vi "流量计.vi"() -> ()   [LabVIEW 2016, in "流量计集成.lvlib"]
uses:
  <vilib>/Plasmionique/MB Master/MB_Master_Serial/MB_Master_Serial.lvclass
  C:/Program Files (x86)/National Instruments/LabVIEW 2016/vi.lib/Plasmionique/MB Master/MB_Master/MB_Master.lvclass
  <vilib>/Analysis/baseanly.llb/Mean (DBL).vi
  <vilib>/Utility/config.llb/NI_LVConfig.lvlib
  <vilib>/Analysis/NI_AALBase.lvlib
panel:
  in  "LSS-100X状态查询":bool
  out "流量计通讯 7":bool caption="通讯"
  out "流量计通讯 6":bool caption="通讯"
  out "流量计通讯 5":bool caption="通讯"
  out "流量计通讯 4":bool caption="通讯"
  out "流量计通讯 3":bool caption="通讯"
  out "流量计通讯 2":bool caption="通讯"
  out "流量计通讯":bool caption="通讯"
  in  "baud rate":u32(ring)=9600 caption="波特率" items=["1200"=1200, "2400"=2400, "4800"=4800, "9600"=9600, "19200"=19200, "38400"=38400, "115200"=115200]
  in  "流量计启用 7":bool
  out "流量计类型 7":T1=enum."LS-H600流量计"
  in  "每小时总流量/总累积流量":bool
  out "通信":bool
  in  "释放串口":bool
  in  "打开串口":bool
  out "serial port":refnum<visa-resource-name>="COM10" caption="串口"
  in  "流量计启用 6":bool
  in  "数量 6":u16
  out "流量计类型 6":T1=enum."LSS-100X流量计"
  in  "运行模式":enum16{"按周期模式", "全常规模式"}(ring)=enum."全常规模式"
  in  "流量计启用 5":bool
  in  "数量 5":u16
  out "流量计类型 5":T1=enum."WL1A1明渠流量计"
  in  "流量计启用 4":bool
  in  "数量 4":u16
  out "流量计类型 4":T1=enum."LSH10-1QC流量计"
  out "平均水位":dbl format="%#.2f"
  out "总累积流量":dbl format="%#.2f"
  out "平均流速":dbl format="%#.2f"
  out "总流量":dbl format="%#.2f"
  in  "选项卡控件":T2(tab)
  out "数组":T3[](array[typedef])
  out "数组 2":T4[](array[typedef]) {"累积流量单位" items=["L", "M3", "T", "USG"]; "瞬时流量单位" items=["L/S", "L/M", "L/H", "M3/S", "M3/M", "M3/H", "T/S", "T/M", "T/H", "GPS", "GPM", "GPH"]}
  out "数组 3":T7[](array[typedef])
  out "数组 4":T3[](array[typedef])
  out "数组 5":T3[](array[typedef])
  out "数组 6":T3[](array[typedef])
  out "数组 7":T3[](array[typedef])
  out "MB_Serial session":refnum<class "MB_Master_Serial.lvclass">
  in  "斯坦道功率测流":bool
  in  "流量计启用 3":bool
  in  "数量 3":u16
  out "流量计类型 3":T1=enum."斯坦道功率测流"
  in  "流量计启用 2":bool
  in  "数量 2":u16
  out "流量计类型 2":T1=enum."MGG/KL QC"
  in  "数量":u16
  out "流量计类型":T1
  in  "流量计启用":bool
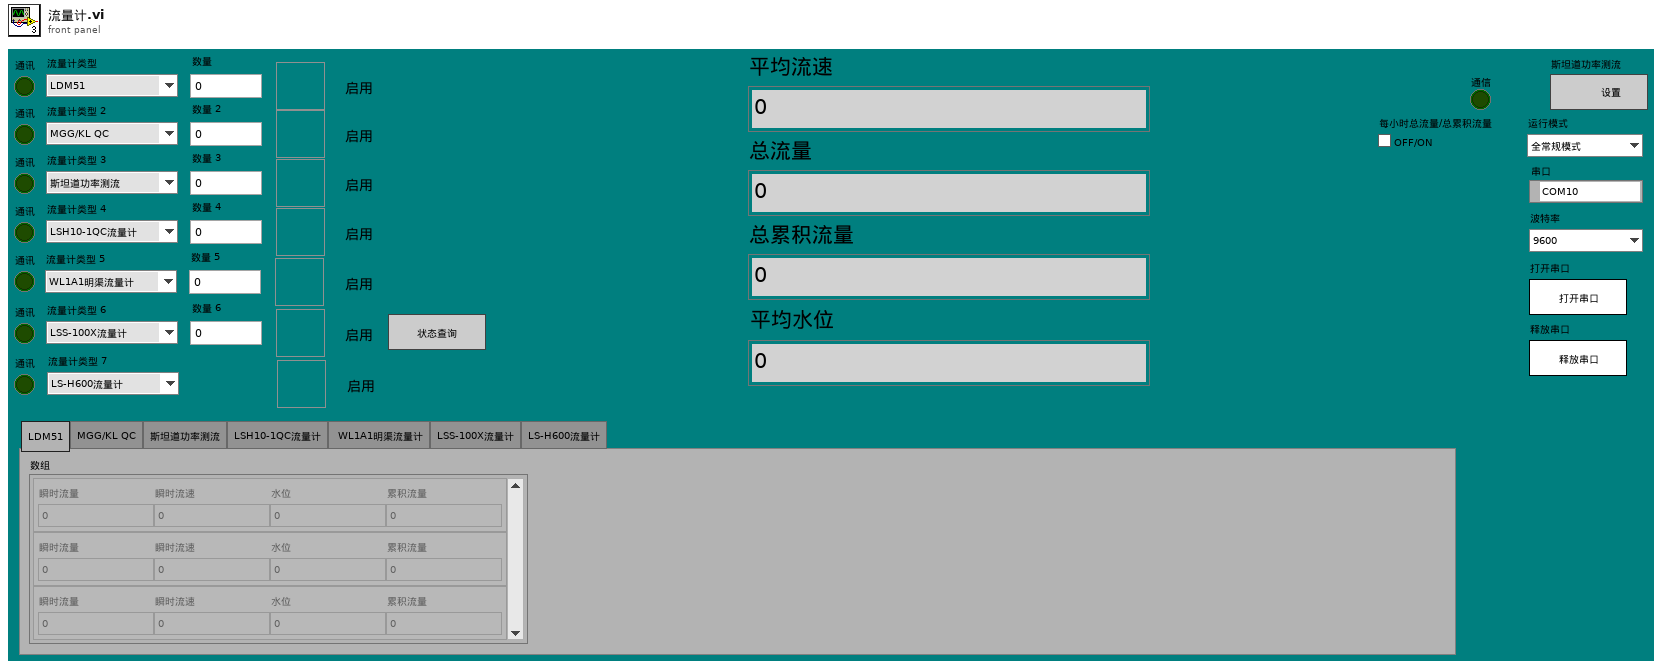
[diagram p1: front panel]
types:
  T1 = typedef "流量计集成.lvlib/流量计类型.ctl" = enum16{"LDM51", "MGG/KL QC", "斯坦道功率测流", "LSH10-1QC流量计", "SL1500-3G", "WL1A1明渠流量计", "LSS-100X流量计", "LS-H600流量计"}
  T2 = enum32{"LDM51", "MGG/KL QC", "斯坦道功率测流", "LSH10-1QC流量计", " WL1A1明渠流量计", "LSS-100X流量计", "LS-H600流量计"}
  T3 = typedef "流量计集成.lvlib/LDM51明渠流量计.lvlib/读取值.ctl" = cluster{"瞬时流量":sgl, "瞬时流速":sgl, "水位":sgl, "累积流量":sgl}
  T4 = typedef "流量计集成.lvlib/MGG-KL-QC流量计.lvlib/读取值.ctl" = cluster{"瞬时流量":sgl, "瞬时流速":sgl, "流量百分比":sgl, "流体电导比":sgl, "正向累积数值":sgl, "反向累积数值":sgl, "瞬时流量单位":T5, "累积流量单位":T6, "上限报警":u16, "下限报警":u16, "空管报警":u16, "系统报警":u16}
  T5 = typedef "流量计集成.lvlib/MGG-KL-QC流量计.lvlib/瞬时流量单位.ctl" = u16
  T6 = typedef "流量计集成.lvlib/MGG-KL-QC流量计.lvlib/累积流量单位.ctl" = u16
  T7 = typedef "流量计集成.lvlib/斯坦道功率测流.lvlib/状态值.ctl" = cluster{"1号瞬时流量":dbl, "2号瞬时流量":dbl, "3号瞬时流量":dbl, "4号瞬时流量":dbl, "5号瞬时流量":dbl, "6号瞬时流量":dbl, "1号累积流量":dbl, "2号累积流量":dbl, "3号累积流量":dbl, "4号累积流量":dbl, "5号累积流量":dbl, "6号累积流量":dbl, "总瞬时流量":dbl, "总累积流量":dbl}
  T8 = typedef "NI_LVConfig.lvlib/Config Data RefNum.ctl" = refnum<k1>
  T9 = cluster{"时间标识":timestamp, "测量模式":string, "数据类型":string, "监测值":sgl, "单位":string, "数据标识":string, "因子编码":string}
  T10 = typedef "LVDateTimeRec.ctl" = cluster{"秒数的小数部分":dbl, "秒":i32, "分":i32, "时":i32, "日":i32, "月":i32, "年":i32, "天数（周）":i32, "天数（年）":i32, "DST":i32}
  T11 = typedef "流量计集成.lvlib/博意达流量计.lvlib/读取值.ctl" = cluster{"瞬时流量":sgl, "瞬时流速":sgl, "水位":sgl, "累积流量":sgl}
  T12 = typedef "流量计集成.lvlib/LSS-100X流量计.lvlib/读取值.ctl" = cluster{"瞬时流量":sgl, "瞬时流速":sgl, "水位":sgl, "累积流量":i32}
  T13 = typedef "流量计集成.lvlib/LS-H600流量计.lvlib/读取值.ctl" = cluster{"瞬时流量":sgl, "瞬时流速":sgl, "水位":sgl, "累积流量":i32}
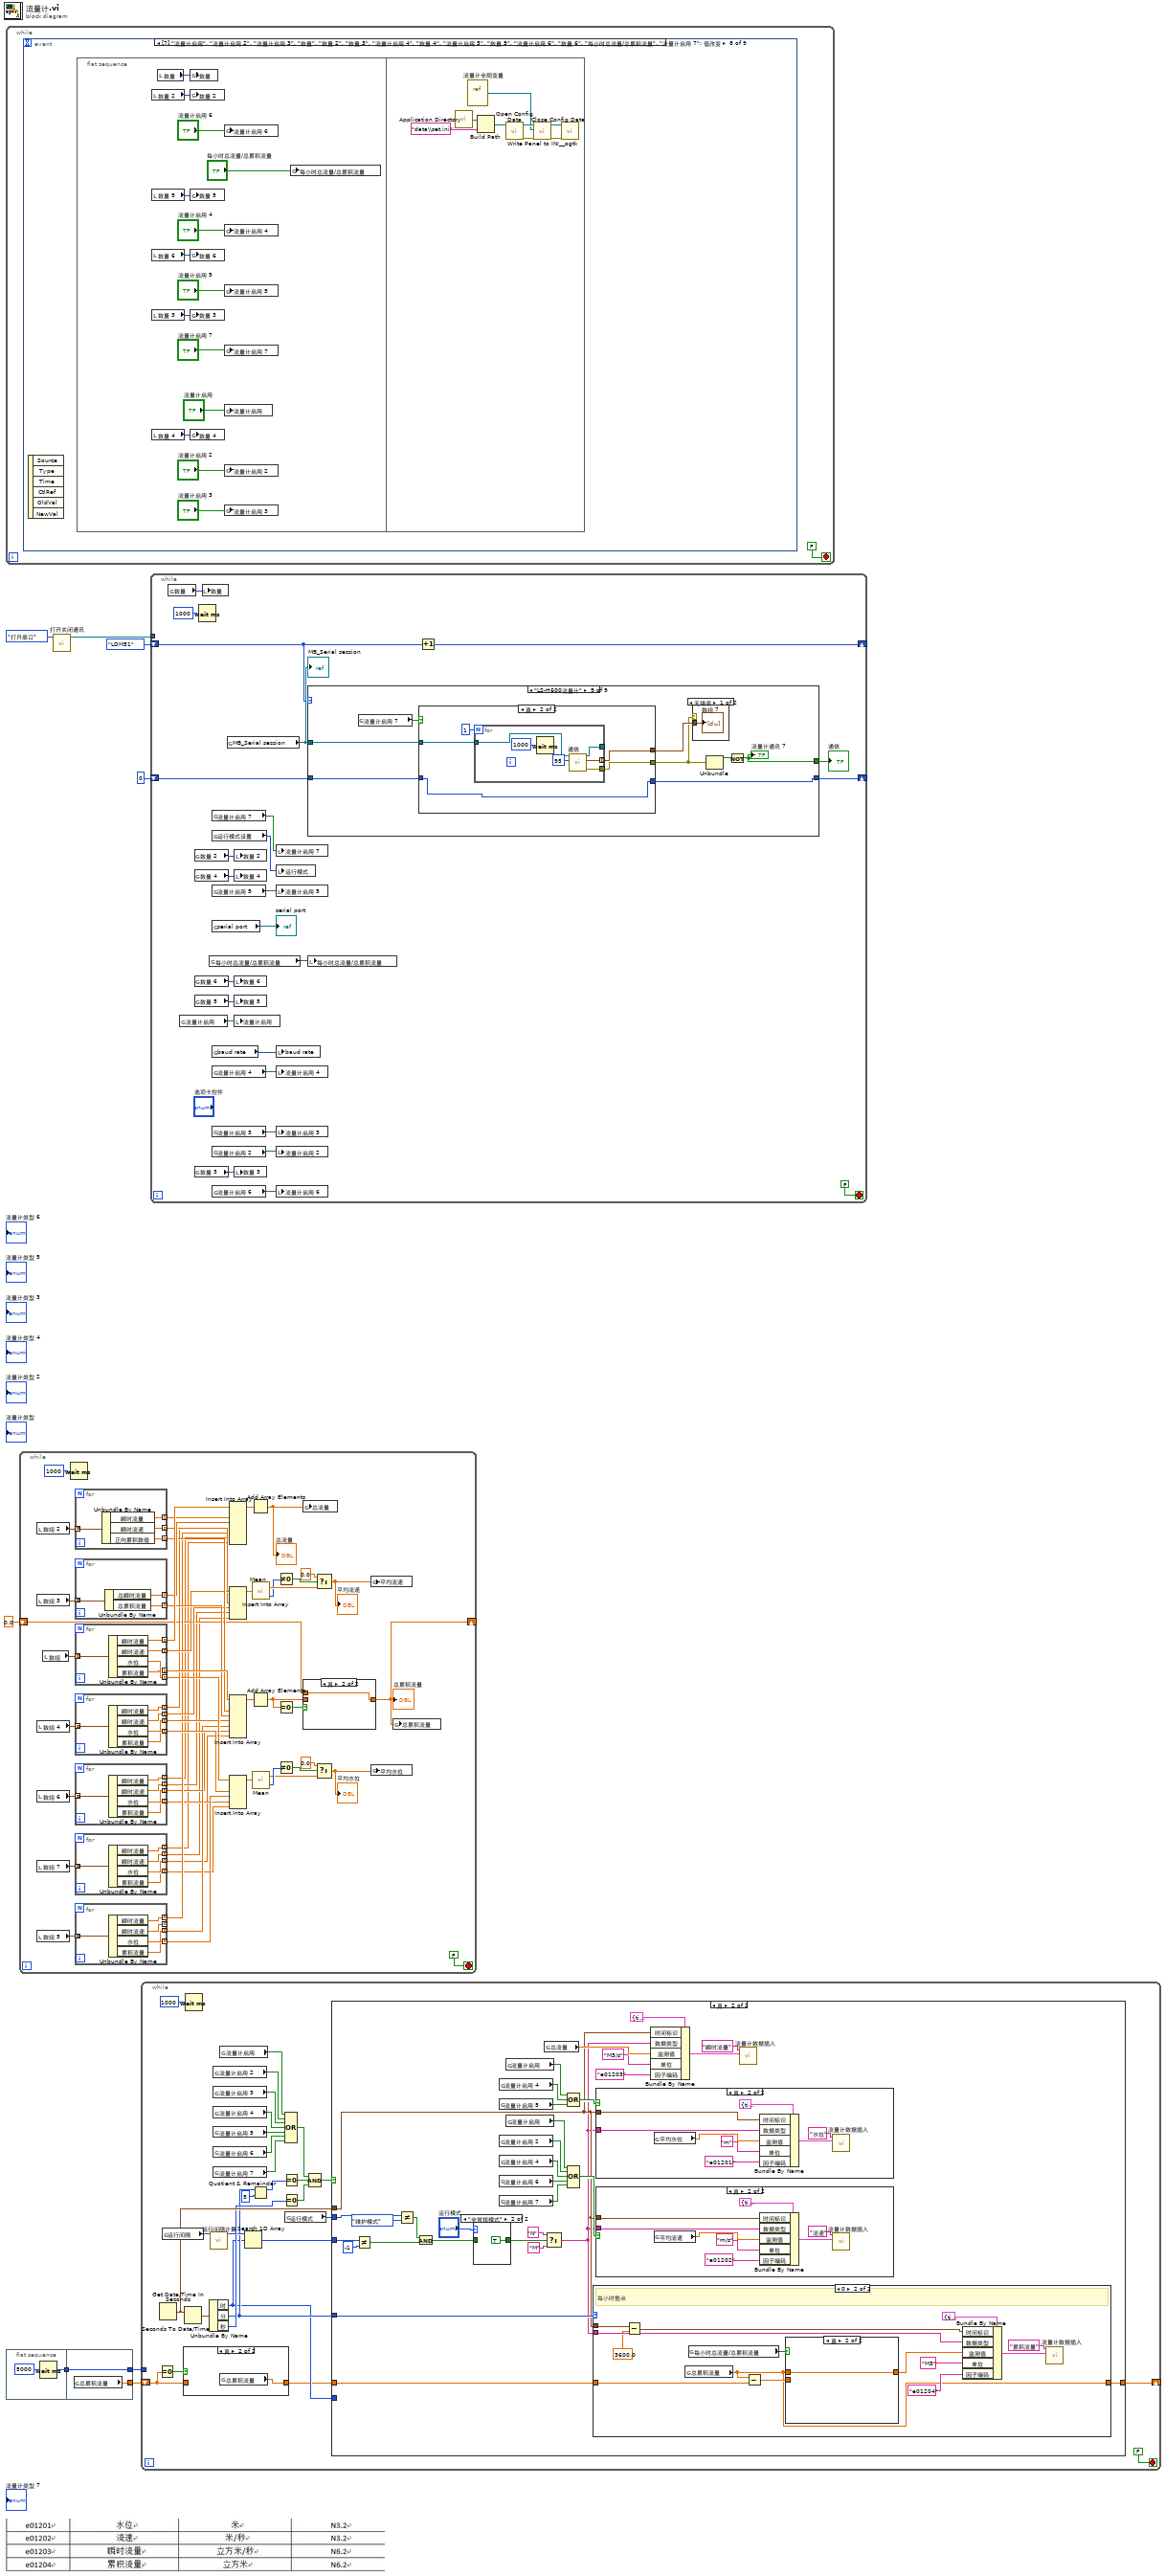
[diagram p0: block diagram]
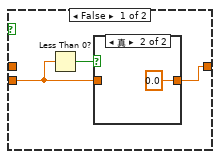
[diagram p6: hidden frame]
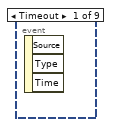
[diagram p11: hidden frame]
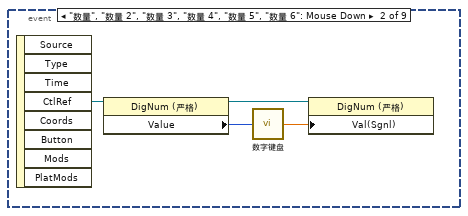
[diagram p12: hidden frame]
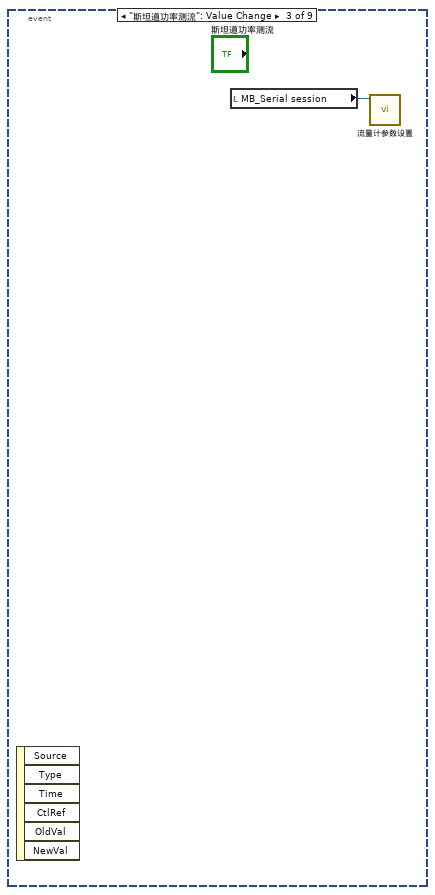
[diagram p13: hidden frame]
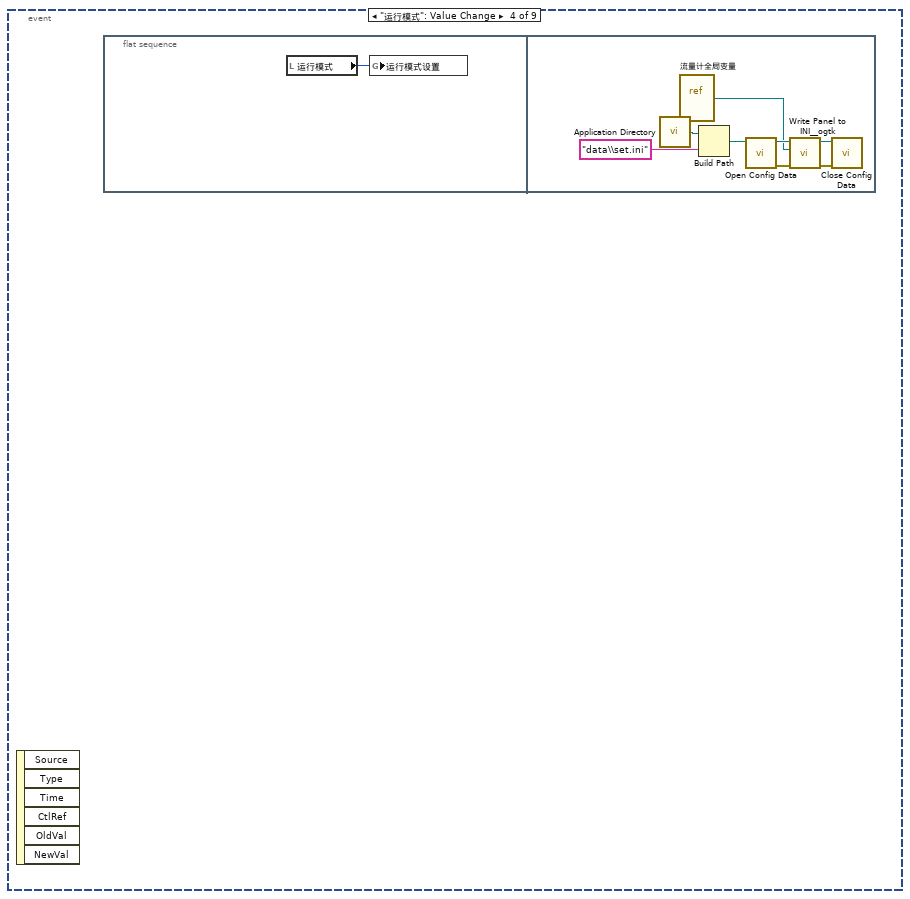
[diagram p14: hidden frame]
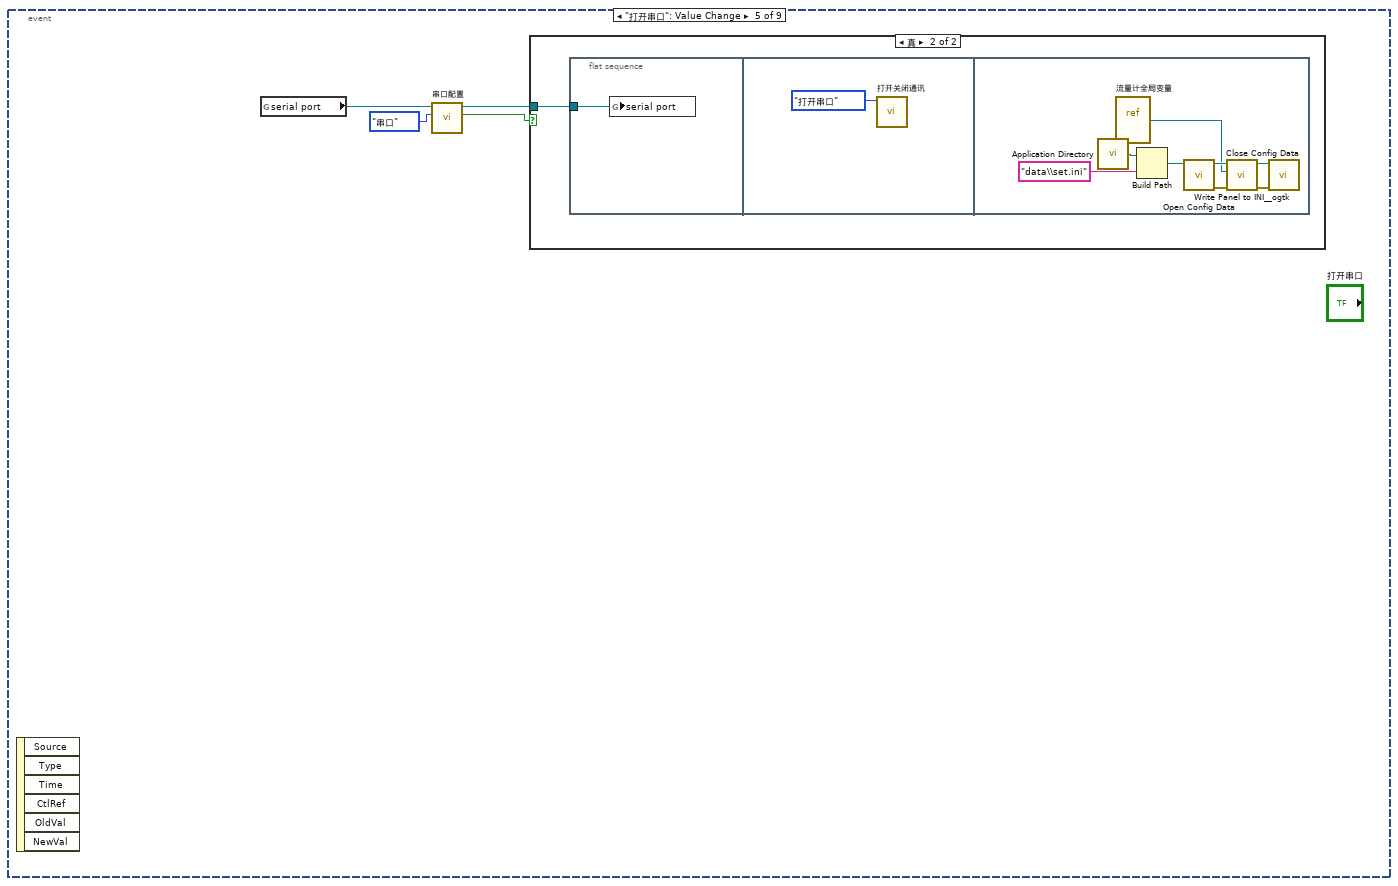
[diagram p15: hidden frame]
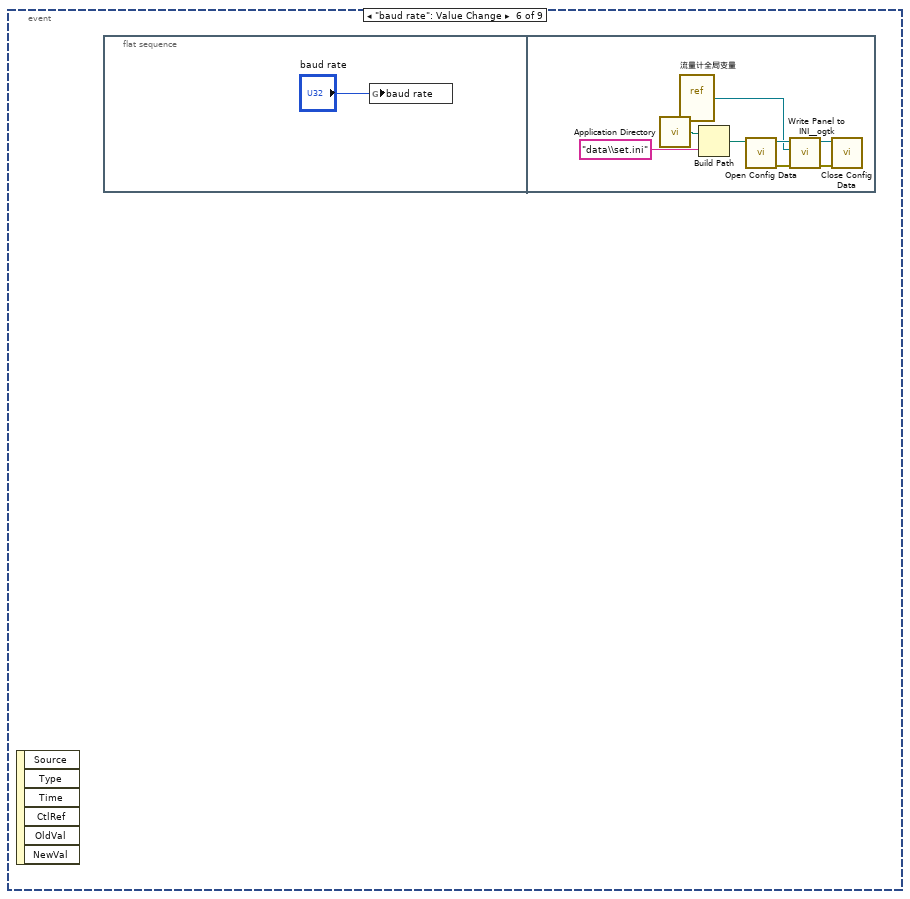
[diagram p17: hidden frame]
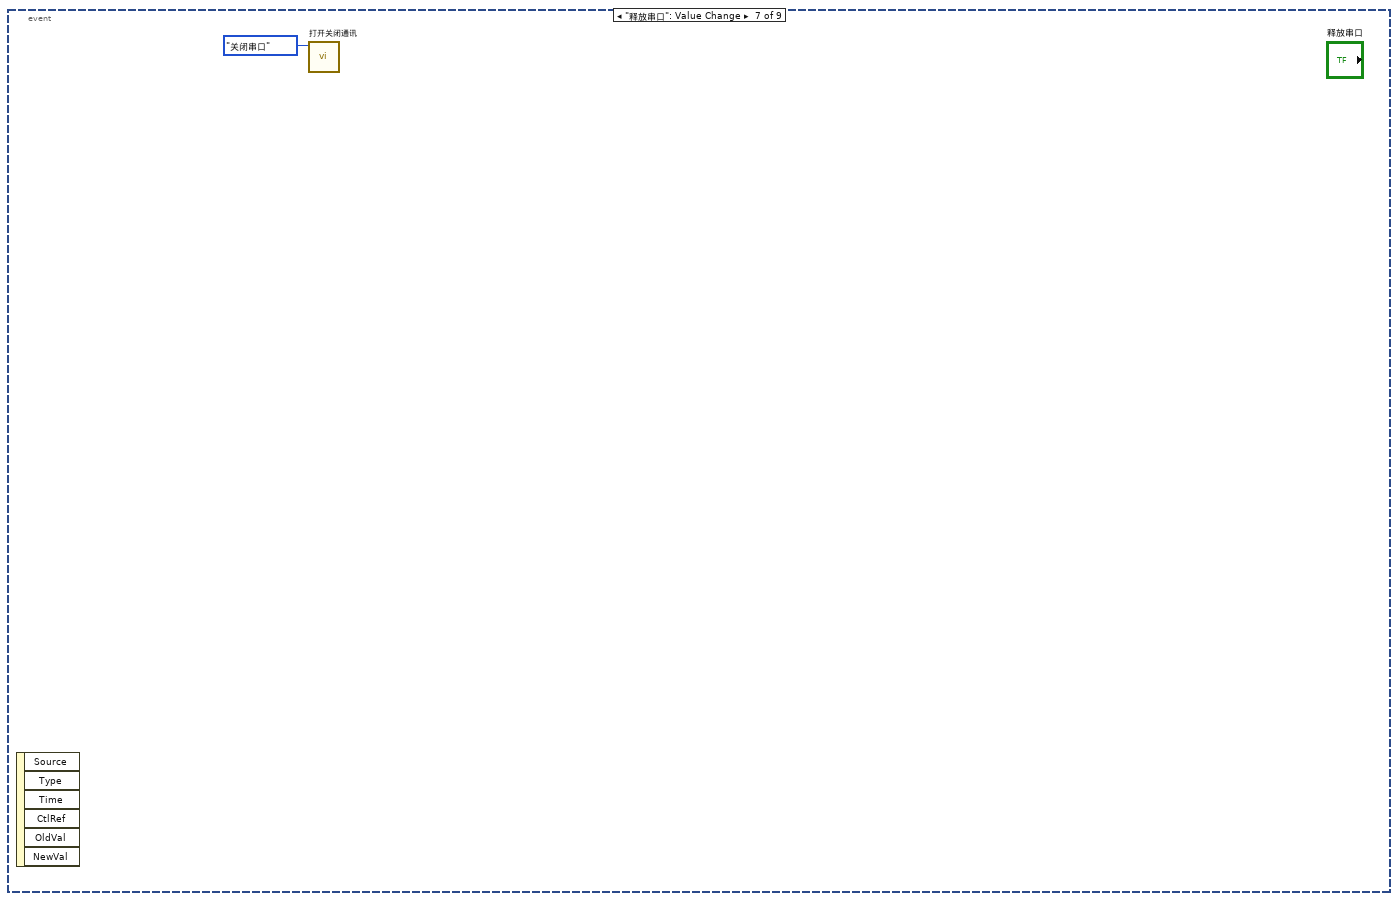
[diagram p18: hidden frame]
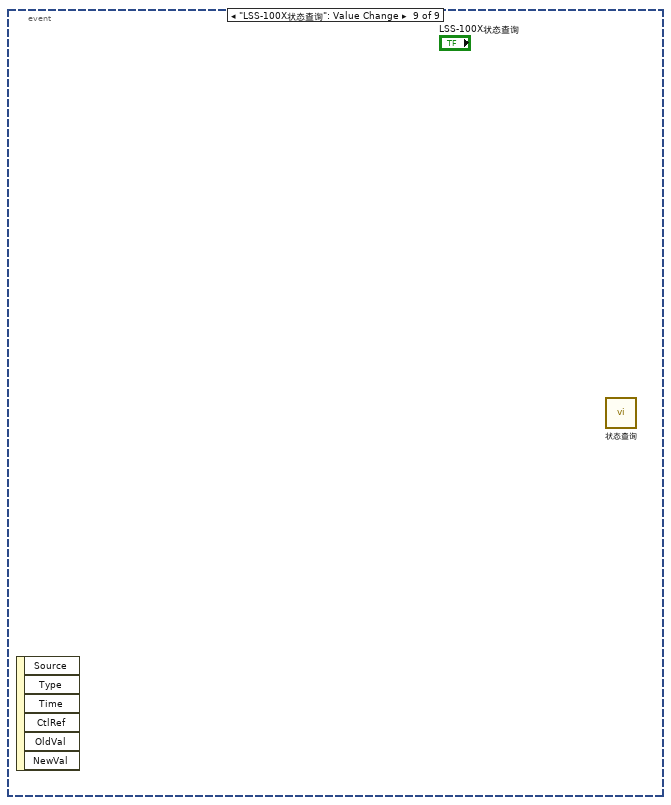
[diagram p19: hidden frame]
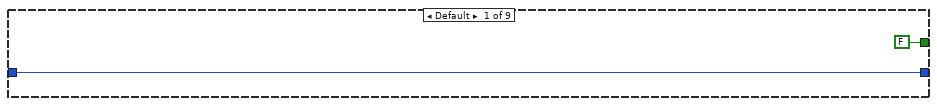
[diagram p20: hidden frame]
diagram:
  n1 = while {
    stop <- FALSE stop-if-true
    n2 = event shown="[7] \"流量计启用\", \"流量计启用 2\", \"流量计启用 3\", \"数量\", \"数量 2\", \"数量 3\", \"流量计启用 4\", \"数量 4\", \"流量计启用 5\", \"数量 5\", \"流量计启用 6\", \"数量 6\", \"每小时总流量/总累积流量\", \"流量计启用 7\": 值改变" {
      selector: _ -> [_ _ _ _ _ _ _ _ _]
      dyn-events: _ -> [_ _ _ _ _ _ _ _ _]
      timeout: _ -> [_ _ _ _ _ _ _ _ _]
      event Timeout {
        n3 = event-data() -> ()  [unwired: 1 in, 3 out]
      }
      event "数量", "数量 2", "数量 3", "数量 4", "数量 5", "数量 6": Mouse Down {
        n4 = event-data() -> ("CtlRef"=w13:refnum<vi>)  [unwired: 1 in, 7 out]
        n5 = property class="DigNum (严格)"(reference=w13) -> (reference out=w11:refnum<vi>, "Value"=w12:u16)  [unwired: 1 in, 1 out]
        n6 = call "数字键盘.vi"("OldNumber"=w12) -> ("NewNumber"=w10:dbl)
        n7 = property class="DigNum (严格)"(reference=w11, "Val(Sgnl)"=w10) -> ()  [unwired: 1 in, 2 out]
      }
      event "斯坦道功率测流": Value Change {
        n8 = event-data() -> ()  [unwired: 1 in, 6 out]
        n9 = local read "MB_Serial session"() -> (w14:refnum<class "MB_Master_Serial.lvclass">)
        n10 = call "流量计参数设置.vi"("MB session in"=w14) -> ()  [unwired: 11 in]
      }
      event "运行模式": Value Change {
        n11 = event-data() -> ()  [unwired: 1 in, 6 out]
        n12 = flat-sequence {
          frame #0 {
            n13 = local read "运行模式"() -> (w15:enum16{"按周期模式", "全常规模式"})
            n14 = global write "流量计全局变量.vi" "运行模式设置"(w15) -> ()
          }
          frame #1 {
            n15 = call <vilib>:"Application Directory.vi"() -> ("Application Directory"=w19:path)
            n16 = vi-ref "流量计全局变量.vi"() -> (w16:refnum<vi>)
            n17 = Build Path(base path=w19, name or relative path="data\\set.ini" ("名称或相对路径")) -> (appended path=w18:path)
            n18 = call <vilib>:"Open Config Data.vi"("configuration file path"=w18) -> ("error out"=w21:errorcluster, "refnum"=w23:T8)  [unwired: 8 in, 1 out]
            n19 = call <userlib>:"Write Panel to INI__ogtk.vi"("error in (no error)"=w21, "VI ref"=w16, "refnum"=w23) -> ("error out"=w20:errorcluster, "refnum out"=w22:T8)  [unwired: 7 in]
            n20 = call <vilib>:"Close Config Data.vi"("error in (no error)"=w20, "refnum"=w22) -> ()  [unwired: 8 in, 2 out]
          }
        }
      }
      event "打开串口": Value Change {
        n21 = event-data() -> ()  [unwired: 1 in, 6 out]
        n22 = global read "流量计全局变量.vi" "serial port"() -> (w26:refnum<visa-resource-name>)
        n23 = call "串口配置.vi"("MB通信方式选择"=enum16{"串口", "TCP"}."串口", "请选择串口:"=w26) -> ("确认 2"=w25:bool, "VISA资源名称 2"=w24:refnum<visa-resource-name>)  [unwired: 5 in, 3 out]
        n24 = case shown="真" w25 {
          tunnel: w24 -> [_ w28]
          frame False {
          }
          frame True {
            n25 = flat-sequence {
              tunnel: w28 -> [w29]
              frame #0 {
                n26 = global write "流量计全局变量.vi" "serial port"(w29) -> ()
              }
              frame #1 {
                n27 = call "打开关闭通讯.vi"("功能输入"=enum16{"打开串口", "关闭串口"}."打开串口") -> ()  [unwired: 9 in, 2 out]
              }
              frame #2 {
                n28 = call <vilib>:"Application Directory.vi"() -> ("Application Directory"=w34:path)
                n29 = vi-ref "流量计全局变量.vi"() -> (w31:refnum<vi>)
                n30 = Build Path(base path=w34, name or relative path="data\\set.ini" ("名称或相对路径")) -> (appended path=w33:path)
                n31 = call <vilib>:"Open Config Data.vi"("configuration file path"=w33) -> ("error out"=w36:errorcluster, "refnum"=w38:T8)  [unwired: 8 in, 1 out]
                n32 = call <userlib>:"Write Panel to INI__ogtk.vi"("error in (no error)"=w36, "VI ref"=w31, "refnum"=w38) -> ("error out"=w35:errorcluster, "refnum out"=w37:T8)  [unwired: 7 in]
                n33 = call <vilib>:"Close Config Data.vi"("error in (no error)"=w35, "refnum"=w37) -> ()  [unwired: 8 in, 2 out]
              }
            }
          }
        }
      }
      event "baud rate": Value Change {
        n34 = event-data() -> ()  [unwired: 1 in, 6 out]
        n35 = flat-sequence {
          frame #0 {
            n36 = global write "流量计全局变量.vi" "baud rate"("baud rate") -> ()
          }
          frame #1 {
            n37 = call <vilib>:"Application Directory.vi"() -> ("Application Directory"=w43:path)
            n38 = vi-ref "流量计全局变量.vi"() -> (w40:refnum<vi>)
            n39 = Build Path(base path=w43, name or relative path="data\\set.ini" ("名称或相对路径")) -> (appended path=w42:path)
            n40 = call <vilib>:"Open Config Data.vi"("configuration file path"=w42) -> ("error out"=w45:errorcluster, "refnum"=w47:T8)  [unwired: 8 in, 1 out]
            n41 = call <userlib>:"Write Panel to INI__ogtk.vi"("error in (no error)"=w45, "VI ref"=w40, "refnum"=w47) -> ("error out"=w44:errorcluster, "refnum out"=w46:T8)  [unwired: 7 in]
            n42 = call <vilib>:"Close Config Data.vi"("error in (no error)"=w44, "refnum"=w46) -> ()  [unwired: 8 in, 2 out]
          }
        }
      }
      event "释放串口": Value Change {
        n43 = event-data() -> ()  [unwired: 1 in, 6 out]
        n44 = call "打开关闭通讯.vi"("功能输入"=enum16{"打开串口", "关闭串口"}."关闭串口") -> ()  [unwired: 9 in, 2 out]
      }
      event "流量计启用", "流量计启用 2", "流量计启用 3", "数量", "数量 2", "数量 3", "流量计启用 4", "数量 4", "流量计启用 5", "数量 5", "流量计启用 6", "数量 6", "每小时总流量/总累积流量", "流量计启用 7": Value Change {
        n45 = event-data() -> ()  [unwired: 1 in, 6 out]
        n46 = flat-sequence {
          frame #0 {
            n47 = local read "数量 2"() -> (w58:u16)
            n48 = local read "数量 5"() -> (w53:u16)
            n49 = local read "数量 6"() -> (w52:u16)
            n50 = local read "数量 3"() -> (w57:u16)
            n51 = local read "数量 4"() -> (w55:u16)
            n52 = local read "数量"() -> (w59:u16)
            n53 = global write "流量计全局变量.vi" "数量"(w59) -> ()
            n54 = global write "流量计全局变量.vi" "数量 2"(w58) -> ()
            n55 = global write "流量计全局变量.vi" "数量 5"(w53) -> ()
            n56 = global write "流量计全局变量.vi" "数量 6"(w52) -> ()
            n57 = global write "流量计全局变量.vi" "数量 3"(w57) -> ()
            n58 = global write "流量计全局变量.vi" "数量 4"(w55) -> ()
            n59 = global write "流量计全局变量.vi" "流量计启用 6"("流量计启用 6") -> ()
            n60 = global write "流量计全局变量.vi" "流量计启用 4"("流量计启用 4") -> ()
            n61 = global write "流量计全局变量.vi" "流量计启用 5"("流量计启用 5") -> ()
            n62 = global write "流量计全局变量.vi" "流量计启用 7"("流量计启用 7") -> ()
            n63 = global write "流量计全局变量.vi" "流量计启用"("流量计启用") -> ()
            n64 = global write "流量计全局变量.vi" "流量计启用 2"("流量计启用 2") -> ()
            n65 = global write "流量计全局变量.vi" "流量计启用 3"("流量计启用 3") -> ()
            n66 = global write "流量计全局变量.vi" "每小时总流量/总累积流量"("每小时总流量/总累积流量") -> ()
          }
          frame #1 {
            n67 = call <vilib>:"Application Directory.vi"() -> ("Application Directory"=w66:path)
            n68 = vi-ref "流量计全局变量.vi"() -> (w63:refnum<vi>)
            n69 = Build Path(base path=w66, name or relative path="data\\set.ini" ("名称或相对路径")) -> (appended path=w65:path)
            n70 = call <vilib>:"Open Config Data.vi"("configuration file path"=w65) -> ("error out"=w68:errorcluster, "refnum"=w70:T8)  [unwired: 8 in, 1 out]
            n71 = call <userlib>:"Write Panel to INI__ogtk.vi"("error in (no error)"=w68, "VI ref"=w63, "refnum"=w70) -> ("error out"=w67:errorcluster, "refnum out"=w69:T8)  [unwired: 7 in]
            n72 = call <vilib>:"Close Config Data.vi"("error in (no error)"=w67, "refnum"=w69) -> ()  [unwired: 8 in, 2 out]
          }
        }
      }
      event "LSS-100X状态查询": Value Change {
        n73 = event-data() -> ()  [unwired: 1 in, 6 out]
        n74 = call "状态查询.vi"() -> ()  [unwired: 12 in]
      }
    }
  }
  n75 = flat-sequence {
    tunnel: [w71] -> w7
    tunnel: [w74] -> w8
    tunnel: w7 -> [w74]
    tunnel: [w73] -> w6
    frame #0 {
      n76 = Wait (ms)(milliseconds to wait=u32 5000 ("等待时间（毫秒）")) -> (millisecond timer value=w71:u32)
    }
    frame #1 {
      n77 = global read "流量计全局变量.vi" "总累积流量"() -> (w73:dbl)
    }
  }
  n78 = while {
    shift-right: [w85] -> _
    shift-left: 0.0 ("总累积流量") -> [w87]
    stop <- FALSE stop-if-true
    n79 = local read "数组 2"() -> (w123:T4[])
    n80 = local read "数组 3"() -> (w122:T7[])
    n81 = local read "数组 4"() -> (w99:T3[])
    n82 = local read "数组 6"() -> (w84:T3[])
    n83 = local read "数组 7"() -> (w79:T3[])
    n84 = local read "数组 5"() -> (w92:T3[])
    n85 = local read "数组"() -> (w126:T3[])
    n86 = Wait (ms)(milliseconds to wait=u32 1000 ("等待时间（毫秒）")) -> ()  [unwired: 1 out]
    n87 = for {
      tunnel: w123 -> [w155] mode=indexing
      tunnel: [w154] -> w120 mode=indexing
      tunnel: [w153] -> w112 mode=indexing
      tunnel: [w152] -> w117 mode=indexing
      n88 = Unbundle By Name(w155) -> ("瞬时流量"=w154:sgl, "瞬时流速"=w153:sgl, "正向累积数值"=w152:sgl)
    }
    n89 = for {
      tunnel: w122 -> [w151] mode=indexing
      tunnel: [w150] -> w119 mode=indexing
      tunnel: [w149] -> w116 mode=indexing
      n90 = Unbundle By Name(w151) -> ("总瞬时流量"=w150:dbl, "总累积流量"=w149:dbl)
    }
    n91 = for {
      tunnel: w126 -> [w160] mode=indexing
      tunnel: [w159] -> w121 mode=indexing
      tunnel: [w158] -> w113 mode=indexing
      tunnel: [w157] -> w96 mode=indexing
      tunnel: [w156] -> w118 mode=indexing
      n92 = Unbundle By Name(w160) -> ("瞬时流量"=w159:sgl, "瞬时流速"=w158:sgl, "水位"=w157:sgl, "累积流量"=w156:sgl)
    }
    n93 = for {
      tunnel: w99 -> [w148] mode=indexing
      tunnel: [w147] -> w97 mode=indexing
      tunnel: [w146] -> w98 mode=indexing
      tunnel: [w145] -> w94 mode=indexing
      tunnel: [w144] -> w93 mode=indexing
      n94 = Unbundle By Name(w148) -> ("瞬时流量"=w147:sgl, "瞬时流速"=w146:sgl, "水位"=w145:sgl, "累积流量"=w144:sgl)
    }
    n95 = for {
      tunnel: w84 -> [w136] mode=indexing
      tunnel: [w135] -> w80 mode=indexing
      tunnel: [w134] -> w83 mode=indexing
      tunnel: [w133] -> w82 mode=indexing
      tunnel: [w132] -> w81 mode=indexing
      n96 = Unbundle By Name(w136) -> ("瞬时流量"=w135:sgl, "瞬时流速"=w134:sgl, "水位"=w133:sgl, "累积流量"=w132:sgl)
    }
    n97 = for {
      tunnel: w79 -> [w131] mode=indexing
      tunnel: [w130] -> w78 mode=indexing
      tunnel: [w129] -> w75 mode=indexing
      tunnel: [w128] -> w76 mode=indexing
      tunnel: [w127] -> w77 mode=indexing
      n98 = Unbundle By Name(w131) -> ("瞬时流量"=w130:sgl, "瞬时流速"=w129:sgl, "水位"=w128:sgl, "累积流量"=w127:sgl)
    }
    n99 = for {
      tunnel: w92 -> [w143] mode=indexing
      tunnel: [w142] -> w90 mode=indexing
      tunnel: [w141] -> _ mode=indexing
      tunnel: [w140] -> w89 mode=indexing
      tunnel: [w139] -> w91 mode=indexing
      n100 = Unbundle By Name(w143) -> ("瞬时流量"=w142:sgl, "瞬时流速"=w141:sgl, "水位"=w140:sgl, "累积流量"=w139:sgl)
    }
    n101 = Insert Into Array(array=w121, new element #1=w120, new element #2=w119, new element #3=w97, new element #4=w90, new element #5=w80, new element #6=w78) -> (w115:sgl[])  [unwired: 1 in]
    n102 = Insert Into Array(array=w113, new element #1=w112, new element #2=w98, new element #3=w83, new element #4=w75) -> (w107:sgl[])  [unwired: 1 in]
    n103 = Insert Into Array(array=w118, new element #1=w117, new element #2=w116, new element #3=w93, new element #4=w91, new element #5=w81, new element #6=w77) -> (w114:sgl[])  [unwired: 1 in]
    n104 = Insert Into Array(array=w96, new element #1=w94, new element #2=w89, new element #3=w82, new element #4=w76) -> (w95:sgl[])  [unwired: 1 in]
    n105 = Add Array Elements(numeric array=w115) -> (sum=w102:sgl)
    "总流量" <- w102
    n106 = Add Array Elements(numeric array=w114) -> (sum=w86:sgl)
    n107 = call-poly <vilib>:"Mean.vi"("X"=w107) -> ("mean"=w111:dbl, "error"=w108:i32)
    n108 = call-poly <vilib>:"Mean.vi"("X"=w95) -> ("mean"=w103:dbl, "error"=w106:i32)
    n109 = Not Equal To 0?(x=w108) -> (x != 0?=w109:bool)
    n110 = Equal To 0?(x=w86) -> (x = 0?=w88:bool)
    n111 = Not Equal To 0?(x=w106) -> (x != 0?=w105:bool)
    n112 = global write "流量计全局变量.vi" "总流量"(w102) -> ()
    n113 = case shown="真" w88 {
      tunnel: w87 -> [_ w138]
      tunnel: [w137 w138] -> w85
      tunnel: w86 -> [w137 _]
      frame False {
      }
      frame True {
      }
    }
    "总累积流量" <- w85
    n114 = Select(t=0.0, s=w109, f=w111) -> (s? t:f=w101:dbl)
    "平均流速" <- w101
    n115 = Select(t=0.0, s=w105, f=w103) -> (s? t:f=w100:dbl)
    "平均水位" <- w100
    n116 = global write "流量计全局变量.vi" "平均流速"(w101) -> ()
    n117 = global write "流量计全局变量.vi" "平均水位"(w100) -> ()
    n118 = global write "流量计全局变量.vi" "总累积流量"(w85) -> ()
  }
  n119 = call "打开关闭通讯.vi"("功能输入"=enum16{"打开串口", "关闭串口"}."打开串口") -> ("MB_Serial session"=w4:refnum<class "MB_Master_Serial.lvclass">)  [unwired: 9 in, 1 out]
  n120 = while {
    tunnel: w8 -> [_]
    shift-right: [w167] -> _
    shift-left: w6 -> [w164]
    stop <- FALSE stop-if-true
    n121 = Equal To 0?(x=w164) -> (x = 0?=w165:bool)
    n122 = Get Date/Time In Seconds() -> (seconds since 1Jan1904=w187:timestamp)
    n123 = global read "流量计全局变量.vi" "运行间隔"() -> (w171:i16)
    n124 = case shown="真" w165 {
      tunnel: [w189 w190] -> w163
      tunnel: w164 -> [w189 _]
      frame False {
      }
      frame True {
        n125 = global read "流量计全局变量.vi" "总累积流量"() -> (w190:dbl)
      }
    }
    n126 = Seconds To Date/Time(time stamp (now)=w187) -> (date time rec=w186:T10)  [unwired: 1 in]
    n127 = Wait (ms)(milliseconds to wait=u32 1000 ("等待时间（毫秒）")) -> ()  [unwired: 1 out]
    n128 = Unbundle By Name(w186) -> ("时"=w166:i32, "分"=w172:i32, "秒"=w184:i32)
    n129 = call "运行间隔计算.vi"("运行周期"=w171) -> ("数组"=w174:i32[])  [unwired: 10 in]
    n130 = global read "流量计全局变量.vi" "流量计启用 2"() -> (w177:bool)
    n131 = global read "流量计全局变量.vi" "流量计启用 3"() -> (w176:bool)
    n132 = global read "流量计全局变量.vi" "流量计启用 4"() -> (w170:bool)
    n133 = global read "流量计全局变量.vi" "流量计启用 5"() -> (w169:bool)
    n134 = global read "流量计全局变量.vi" "流量计启用 6"() -> (w162:bool)
    n135 = global read "流量计全局变量.vi" "流量计启用 7"() -> (w161:bool)
    n136 = global read "流量计全局变量.vi" "流量计启用"() -> (w178:bool)
    n137 = Search 1D Array(1D array=w174, element=w166) -> (index of element=w173:i32)  [unwired: 1 in]
    n138 = Quotient & Remainder(x=w172, y=5) -> (x-y*floor(x/y)=w183:i32)  [unwired: 1 out]
    n139 = Equal To 0?(x=w183) -> (x = 0?=w182:bool)
    n140 = Equal To 0?(x=w184) -> (x = 0?=w181:bool)
    n141 = Compound Arithmetic op=OR ("复合运算")(w178, w177, w176, w170, w169, w162, w161) -> (w175:bool)
    n142 = global read "流量计全局变量.vi" "运行模式"() -> (w168:enum16{"维护模式", "常规模式", "应急模式", "质控模式", "性能测试"})
    n143 = Compound Arithmetic op=AND ("复合运算")(w175, w182, w181) -> (w180:bool)
    n144 = case shown="真" w180 {
      tunnel: w187 -> [_ w196]
      tunnel: w173 -> [_ w217]
      tunnel: w172 -> [_ w216]
      tunnel: w168 -> [_ w209]
      tunnel: [w191 w204] -> w167
      tunnel: w163 -> [w191 w203]
      tunnel: w166 -> [_ _]
      frame False {
      }
      frame True {
        n145 = Not Equal?(x=w217, y=-1) -> (x != y?=w220:bool)
        n146 = Not Equal?(x=w209, y=enum16{"维护模式", "常规模式", "应急模式", "质控模式", "性能测试"}."维护模式") -> (x != y?=w208:bool)
        n147 = And(x=w208, y=w220) -> (x .and. y?=w206:bool)
        n148 = case shown="\"全常规模式\"" "运行模式" {
          tunnel: w206 -> [w245 _]
          tunnel: [w245 TRUE] -> w205
          frame "按周期模式", Default {
          }
          frame "全常规模式" {
          }
        }
        n149 = global read "流量计全局变量.vi" "流量计启用 4"() -> (w212:bool)
        n150 = global read "流量计全局变量.vi" "流量计启用 5"() -> (w211:bool)
        n151 = global read "流量计全局变量.vi" "流量计启用 2"() -> (w222:bool)
        n152 = global read "流量计全局变量.vi" "流量计启用 4"() -> (w215:bool)
        n153 = global read "流量计全局变量.vi" "流量计启用 6"() -> (w194:bool)
        n154 = global read "流量计全局变量.vi" "流量计启用 7"() -> (w193:bool)
        n155 = global read "流量计全局变量.vi" "流量计启用"() -> (w213:bool)
        n156 = global read "流量计全局变量.vi" "流量计启用"() -> (w223:bool)
        n157 = global read "流量计全局变量.vi" "总流量"() -> (w200:dbl)
        n158 = Select(t="N" ("单位"), s=w205, f="M" ("单位")) -> (s? t:f=w195:string)
        n159 = Compound Arithmetic op=OR ("复合运算")(w213, w212, w211) -> (w210:bool)
        n160 = Compound Arithmetic op=OR ("复合运算")(w223, w222, w215, w194, w193) -> (w214:bool)
        n161 = case shown="0" w216 {
          tunnel: w196 -> [_ w238]
          tunnel: w195 -> [_ w236]
          tunnel: [w224 w227] -> w204
          tunnel: w203 -> [w224 w231]
          frame Default {
          }
          frame 0 {
            # "每小时整点"
            n162 = Subtract(x=w238, y=3600.0) -> (x-y=w225:timestamp)
            n163 = global read "流量计全局变量.vi" "总累积流量"() -> (w227:dbl)
            n164 = global read "流量计全局变量.vi" "每小时总流量/总累积流量"() -> (w228:bool)
            n165 = Subtract(x=w227, y=w231) -> (x-y=w229:dbl)
            n166 = case shown="真" w228 {
              tunnel: [w240 w244] -> w230
              tunnel: w229 -> [w239 _]
              tunnel: w227 -> [_ w244]
              frame False {
                n167 = Less Than 0?(x=w239) -> (x < 0?=w241:bool)
                n168 = case shown="真" w241 {
                  tunnel: [w242 0.0] -> w240
                  tunnel: w239 -> [w242 _]
                  frame False {
                  }
                  frame True {
                  }
                }
              }
              frame True {
              }
            }
            n169 = Bundle By Name(cluster=T9 {"时间标识"=timestamp(0 s since 1904-01-01), "测量模式"="水样测试", "数据类型"="N", "监测值"=0.0, "单位"="mg/L", "数据标识"="N", "因子编码"=""} ("data"), "时间标识"=w225, "数据类型"=w236, "监测值"=w230, "单位"="M3", "因子编码"="e01204") -> (w233:T9)
            n170 = call "流量计数据插入.vi"("Tabe Name"="累积流量" ("table 输入"), "data"=w233) -> ()  [unwired: 8 in, 1 out]
          }
        }
        n171 = case shown="真" w210 {
          tunnel: w196 -> [_ w251]
          tunnel: w195 -> [_ w250]
          frame False {
          }
          frame True {
            n172 = global read "流量计全局变量.vi" "平均水位"() -> (w249:dbl)
            n173 = Bundle By Name(cluster=T9 {"时间标识"=timestamp(0 s since 1904-01-01), "测量模式"="水样测试", "数据类型"="N", "监测值"=0.0, "单位"="mg/L", "数据标识"="N", "因子编码"=""} ("data"), "时间标识"=w251, "数据类型"=w250, "监测值"=w249, "单位"="m", "因子编码"="e01201") -> (w248:T9)
            n174 = call "流量计数据插入.vi"("Tabe Name"="水位" ("table 输入"), "data"=w248) -> ()  [unwired: 8 in, 1 out]
          }
        }
        n175 = case shown="真" w214 {
          tunnel: w196 -> [_ w258]
          tunnel: w195 -> [_ w257]
          frame False {
          }
          frame True {
            n176 = global read "流量计全局变量.vi" "平均流速"() -> (w259:dbl)
            n177 = Bundle By Name(cluster=T9 {"时间标识"=timestamp(0 s since 1904-01-01), "测量模式"="水样测试", "数据类型"="N", "监测值"=0.0, "单位"="mg/L", "数据标识"="N", "因子编码"=""} ("data"), "时间标识"=w258, "数据类型"=w257, "监测值"=w259, "单位"="m/s", "因子编码"="e01202") -> (w255:T9)
            n178 = call "流量计数据插入.vi"("Tabe Name"="流速" ("table 输入"), "data"=w255) -> ()  [unwired: 8 in, 1 out]
          }
        }
        n179 = Bundle By Name(cluster=T9 {"时间标识"=timestamp(0 s since 1904-01-01), "测量模式"="水样测试", "数据类型"="N", "监测值"=0.0, "单位"="mg/L", "数据标识"="N", "因子编码"=""} ("data"), "时间标识"=w196, "数据类型"=w195, "监测值"=w200, "单位"="M3/s", "因子编码"="e01203") -> (w198:T9)
        n180 = call "流量计数据插入.vi"("Tabe Name"="瞬时流量" ("table 输入"), "data"=w198) -> ()  [unwired: 8 in, 1 out]
      }
    }
  }
  n181 = while {
    tunnel: w4 -> [_]
    shift-right: [w266] -> _
    shift-left: 流量计类型."LDM51" ("流量计类型") -> [w267]
    shift-right: [w263] -> _
    shift-left: u16 0 ("数量") -> [w264]
    stop <- FALSE stop-if-true
    n182 = global read "流量计全局变量.vi" "数量"() -> (w285:u16)
    n183 = global read "流量计全局变量.vi" "流量计启用"() -> (w274:bool)
    n184 = global read "流量计全局变量.vi" "数量 2"() -> (w284:u16)
    n185 = global read "流量计全局变量.vi" "数量 4"() -> (w282:u16)
    n186 = global read "流量计全局变量.vi" "数量 6"() -> (w280:u16)
    n187 = global read "流量计全局变量.vi" "数量 5"() -> (w279:u16)
    n188 = global read "流量计全局变量.vi" "数量 3"() -> (w283:u16)
    n189 = Wait (ms)(milliseconds to wait=u32 1000 ("等待时间（毫秒）")) -> ()  [unwired: 1 out]
    n190 = local write "数量"(w285) -> ()
    n191 = global read "流量计全局变量.vi" "每小时总流量/总累积流量"() -> (w276:bool)
    n192 = global read "流量计全局变量.vi" "流量计启用 7"() -> (w268:bool)
    n193 = global read "流量计全局变量.vi" "运行模式设置"() -> (w281:enum16{"按周期模式", "全常规模式"})
    n194 = global read "流量计全局变量.vi" "流量计启用 5"() -> (w270:bool)
    n195 = global read "流量计全局变量.vi" "serial port"() -> (→"serial port":refnum<visa-resource-name>)
    n196 = global read "流量计全局变量.vi" "baud rate"() -> (w275:u32)
    n197 = global read "流量计全局变量.vi" "流量计启用 4"() -> (w271:bool)
    n198 = global read "流量计全局变量.vi" "流量计启用 3"() -> (w272:bool)
    n199 = global read "流量计全局变量.vi" "流量计启用 2"() -> (w273:bool)
    n200 = global read "流量计全局变量.vi" "流量计启用 6"() -> (w269:bool)
    n201 = global read "流量计全局变量.vi" "MB_Serial session"() -> (w278:refnum<class "MB_Master_Serial.lvclass">)
    "MB_Serial session" <- w278
    n202 = local write "数量 2"(w284) -> ()
    n203 = local write "数量 4"(w282) -> ()
    n204 = local write "数量 6"(w280) -> ()
    n205 = local write "数量 5"(w279) -> ()
    n206 = local write "流量计启用"(w274) -> ()
    n207 = local write "数量 3"(w283) -> ()
    n208 = local write "流量计启用 7"(w268) -> ()
    n209 = local write "运行模式"(w281) -> ()
    n210 = local write "流量计启用 5"(w270) -> ()
    n211 = local write "baud rate"(w275) -> ()
    n212 = local write "流量计启用 4"(w271) -> ()
    n213 = local write "流量计启用 3"(w272) -> ()
    n214 = local write "流量计启用 2"(w273) -> ()
    n215 = local write "流量计启用 6"(w269) -> ()
    n216 = case shown="\"LS-H600流量计\"" w267 {
      tunnel: w278 -> [_ w296 w317 w340 w361 _ w388 w413 w439]
      tunnel: [FALSE w293 w314 w338 w359 FALSE w386 w411 w437] -> w265
      tunnel: w264 -> [w288 w292 w313 w337 w358 w381 w385 w410 w435]
      tunnel: [w288 w291 w312 w337 w357 w381 w384 w409 w436] -> w263
      frame Default {
      }
      frame "LDM51" {
        n217 = global read "流量计全局变量.vi" "流量计启用"() -> (w297:bool)
        n218 = case shown="真" w297 {
          tunnel: w296 -> [_ w304]
          tunnel: [_ w303] -> w295
          tunnel: [errorcluster {"status"=TRUE, "code"=0, "source"=""} ("error out") w302] -> w290
          tunnel: w292 -> [_ _]
          tunnel: [u16 0 ("数量") "数量"] -> w291
          frame False {
          }
          frame True {
            n219 = for {
              N: "数量" -> [_]
              tunnel: w304 -> [w310]
              tunnel: [w309] -> w302
              tunnel: [w306] -> w303 mode=indexing
              i -> [w308]
              n220 = Increment(x=w308) -> (x+1=w307:i32)
              n221 = Wait (ms)(milliseconds to wait=u32 1000 ("等待时间（毫秒）")) -> ()  [unwired: 1 out]
              n222 = call "读取数值.vi"("Slave ID"=w307, "MB session in"=w310) -> ("error out"=w309:errorcluster, "读取值"=w306:T3)  [unwired: 7 in, 1 out]
            }
          }
        }
        n223 = Unbundle(w290) -> ("status"=w294:bool)  [unwired: 2 out]
        n224 = case shown="无错误" w290 {
          tunnel: w295 -> [w298 _]
          frame No Error {
            "数组" <- w298
          }
          frame Error {
          }
        }
        n225 = Not(x=w294) -> (.not. x?=w293:bool)
        "流量计通讯" <- w293
      }
      frame "MGG/KL QC" {
        n226 = global read "流量计全局变量.vi" "流量计启用 2"() -> (w318:bool)
        n227 = case shown="真" w318 {
          tunnel: w317 -> [_ w327]
          tunnel: [_ w326] -> w316
          tunnel: [errorcluster {"status"=TRUE, "code"=0, "source"=""} ("error out") w325] -> w311
          tunnel: w313 -> [w320 w324]
          tunnel: [w320 w322] -> w312
          frame False {
          }
          frame True {
            n228 = for {
              N: "数量 2" -> [_]
              tunnel: w327 -> [w334]
              tunnel: w324 -> [w331]
              tunnel: [w330] -> w326 mode=indexing
              tunnel: [w329] -> w325
              i -> [w332]
              n229 = Add(x=w332, y=w331) -> (x+y=w333:i32)
              n230 = Wait (ms)(milliseconds to wait=u32 1000 ("等待时间（毫秒）")) -> ()  [unwired: 1 out]
              n231 = Increment(x=w333) -> (x+1=w335:i32)
              n232 = call "读取数据.vi"("Slave ID"=w335, "MB session in"=w334) -> ("error out"=w329:errorcluster, "读取值"=w330:T4)  [unwired: 6 in, 2 out]
            }
            n233 = Add(x=w324, y="数量 2") -> (x+y=w322:u16)
          }
        }
        n234 = case shown="无错误" w311 {
          tunnel: w316 -> [w319 _]
          frame No Error {
            "数组 2" <- w319
          }
          frame Error {
          }
        }
        n235 = Unbundle(w311) -> ("status"=w315:bool)  [unwired: 2 out]
        n236 = Not(x=w315) -> (.not. x?=w314:bool)
        "流量计通讯 2" <- w314
      }
      frame "斯坦道功率测流" {
        n237 = global read "流量计全局变量.vi" "流量计启用 3"() -> (w342:bool)
        n238 = case shown="真" w342 {
          tunnel: [_ w347] -> w341
          tunnel: [errorcluster {"status"=TRUE, "code"=0, "source"=""} ("error out") w346] -> w336
          tunnel: w340 -> [_ w345]
          frame False {
          }
          frame True {
            n239 = for {
              N: "数量 3" -> [_]
              tunnel: [w352] -> w346
              tunnel: [w351] -> w347 mode=indexing
              tunnel: w345 -> [w349]
              i -> [w355]
              n240 = Add(x=w355, y=20) -> (x+y=w353:i32)
              n241 = Wait (ms)(milliseconds to wait=u32 1000 ("等待时间（毫秒）")) -> ()  [unwired: 1 out]
              n242 = call "读取状态值.vi"("Slave ID"=w353, "MB session in"=w349) -> ("error out"=w352:errorcluster, "状态值"=w351:T7)  [unwired: 6 in, 2 out]
            }
          }
        }
        n243 = case shown="无错误" w336 {
          tunnel: w341 -> [w343 _]
          frame No Error {
            "数组 3" <- w343
          }
          frame Error {
          }
        }
        n244 = Unbundle(w336) -> ("status"=w339:bool)  [unwired: 2 out]
        n245 = Not(x=w339) -> (.not. x?=w338:bool)
        "流量计通讯 3" <- w338
      }
      frame "LSH10-1QC流量计" {
        n246 = global read "流量计全局变量.vi" "流量计启用 4"() -> (w363:bool)
        n247 = case shown="真" w363 {
          tunnel: [_ w372] -> w362
          tunnel: w361 -> [_ w371]
          tunnel: [errorcluster {"status"=TRUE, "code"=0, "source"=""} ("error out") w370] -> w356
          tunnel: w358 -> [w365 w369]
          tunnel: [w365 w367] -> w357
          frame False {
          }
          frame True {
            n248 = for {
              N: "数量 4" -> [_]
              tunnel: [w380] -> w370
              tunnel: [w379] -> w372 mode=indexing
              tunnel: w371 -> [w375]
              tunnel: w369 -> [w373]
              i -> [w377]
              n249 = Add(x=w373, y=w377) -> (x+y=w374:i32)
              n250 = Wait (ms)(milliseconds to wait=u32 1000 ("等待时间（毫秒）")) -> ()  [unwired: 1 out]
              n251 = Increment(x=w374) -> (x+1=w376:i32)
              n252 = call "读取数值.vi"("Slave ID"=w376, "MB session in"=w375) -> ("error out"=w380:errorcluster, "读取值"=w379:T11)  [unwired: 7 in, 1 out]
            }
            n253 = Add(x=w369, y="数量 4") -> (x+y=w367:u16)
          }
        }
        n254 = case shown="无错误" w356 {
          tunnel: w362 -> [w364 _]
          frame No Error {
            "数组 4" <- w364
          }
          frame Error {
          }
        }
        n255 = Unbundle(w356) -> ("status"=w360:bool)  [unwired: 2 out]
        n256 = Not(x=w360) -> (.not. x?=w359:bool)
        "流量计通讯 4" <- w359
      }
      frame "SL1500-3G" {
      }
      frame "WL1A1明渠流量计" {
        n257 = global read "流量计全局变量.vi" "流量计启用 5"() -> (w390:bool)
        n258 = case shown="真" w390 {
          tunnel: [_ w399] -> w389
          tunnel: w388 -> [_ w398]
          tunnel: [errorcluster {"status"=TRUE, "code"=0, "source"=""} ("error out") w397] -> w383
          tunnel: w385 -> [w392 w396]
          tunnel: [w392 w394] -> w384
          frame False {
          }
          frame True {
            n259 = for {
              N: "数量 5" -> [_]
              tunnel: [w404] -> w399 mode=indexing
              tunnel: [w403] -> w397
              tunnel: w398 -> [w402]
              tunnel: w396 -> [w400]
              i -> [w406]
              n260 = Add(x=w406, y=w400) -> (x+y=w401:i32)
              n261 = Wait (ms)(milliseconds to wait=u32 1000 ("等待时间（毫秒）")) -> ()  [unwired: 1 out]
              n262 = Increment(x=w401) -> (x+1=w405:i32)
              n263 = call "读取数值.vi"("Slave ID"=w405, "MB session in"=w402) -> ("error out"=w403:errorcluster, "读取值"=w404:T11)  [unwired: 7 in, 1 out]
            }
            n264 = Add(x=w396, y="数量 5") -> (x+y=w394:u16)
          }
        }
        n265 = case shown="无错误" w383 {
          tunnel: w389 -> [w391 _]
          frame No Error {
            "数组 5" <- w391
          }
          frame Error {
          }
        }
        n266 = Unbundle(w383) -> ("status"=w387:bool)  [unwired: 2 out]
        n267 = Not(x=w387) -> (.not. x?=w386:bool)
        "流量计通讯 5" <- w386
      }
      frame "LSS-100X流量计" {
        n268 = global read "流量计全局变量.vi" "流量计启用 6"() -> (w414:bool)
        n269 = case shown="真" w414 {
          tunnel: [_ w424] -> w415
          tunnel: w413 -> [_ w423]
          tunnel: [errorcluster {"status"=TRUE, "code"=0, "source"=""} ("error out") w422] -> w408
          tunnel: w410 -> [w417 w421]
          tunnel: [w417 w419] -> w409
          frame False {
          }
          frame True {
            n270 = for {
              N: "数量 6" -> [_]
              tunnel: [w430] -> _
              tunnel: [w429] -> w424 mode=indexing
              tunnel: [w428] -> w422
              tunnel: w423 -> [w427]
              tunnel: w421 -> [w425]
              i -> [w432]
              n271 = Add(x=w425, y=w432) -> (x+y=w426:i32)
              n272 = Wait (ms)(milliseconds to wait=u32 1000 ("等待时间（毫秒）")) -> ()  [unwired: 1 out]
              n273 = Increment(x=w426) -> (x+1=w431:i32)
              n274 = call "通信.vi"("Slave ID"=w431, "MB session in"=w427) -> ("error out"=w428:errorcluster, "读取值"=w429:T12, "MB session out"=w430:refnum<class "MB_Master_Serial.lvclass">)  [unwired: 7 in]
            }
            n275 = Add(x=w421, y="数量 6") -> (x+y=w419:u16)
          }
        }
        n276 = case shown="无错误" w408 {
          tunnel: w415 -> [w416 _]
          frame No Error {
            "数组 6" <- w416
          }
          frame Error {
          }
        }
        n277 = Unbundle(w408) -> ("status"=w412:bool)  [unwired: 2 out]
        n278 = Not(x=w412) -> (.not. x?=w411:bool)
        "流量计通讯 6" <- w411
      }
      frame "LS-H600流量计" {
        n279 = global read "流量计全局变量.vi" "流量计启用 7"() -> (w440:bool)
        n280 = case shown="真" w440 {
          tunnel: [_ w449] -> w441
          tunnel: [errorcluster {"status"=TRUE, "code"=0, "source"=""} ("error out") w448] -> w434
          tunnel: w439 -> [_ w447]
          tunnel: [w443 w445] -> w436
          tunnel: w435 -> [w443 w445]
          frame False {
          }
          frame True {
            n281 = for {
              N: 1 -> [_]
              tunnel: [w453] -> _
              tunnel: [w452] -> w449 mode=indexing
              tunnel: [w454] -> w448
              tunnel: w447 -> [w451]
              n282 = Wait (ms)(milliseconds to wait=u32 1000 ("等待时间（毫秒）")) -> ()  [unwired: 1 out]
              n283 = call "通信.vi"("Slave ID"=u8 95, "MB session in"=w451) -> ("error out"=w454:errorcluster, "读取值"=w452:T13, "MB session out"=w453:refnum<class "MB_Master_Serial.lvclass">)  [unwired: 7 in]
            }
          }
        }
        n284 = case shown="无错误" w434 {
          tunnel: w441 -> [w442 _]
          frame No Error {
            "数组 7" <- w442
          }
          frame Error {
          }
        }
        n285 = Unbundle(w434) -> ("status"=w438:bool)  [unwired: 2 out]
        n286 = Not(x=w438) -> (.not. x?=w437:bool)
        "流量计通讯 7" <- w437
      }
    }
    "通信" <- w265
    n287 = local write "每小时总流量/总累积流量"(w276) -> ()
    n288 = Increment(x=w267) -> (x+1=w266:T1)
  }
